vi "PhotonVision_PoseEstData_Alternate.vi"() -> ()   [LabVIEW 2019]
uses:
  <vilib>/Rock Robotics/WPI/ThirdParty/PhotonPoseStrategy_ENUM.ctl
  <vilib>/Rock Robotics/WPI/ThirdParty/PhotonVisionLib/TypeDef/PhotonEstimatedRobotPoseType.ctl
  <vilib>/Rock Robotics/WPI/ThirdParty/JAS_Junk/TrajLib/TypeDef/POSE3D.ctl
  <vilib>/Rock Robotics/WPI/ThirdParty/JAS_Junk/TrajLib/TypeDef/TRANSLATION3D.ctl
  <vilib>/Rock Robotics/WPI/ThirdParty/JAS_Junk/TrajLib/TypeDef/ROTATION3D.ctl
  <vilib>/Rock Robotics/WPI/ThirdParty/JAS_Junk/TrajLib/TypeDef/QUATERNION.ctl
  <vilib>/Rock Robotics/WPI/ThirdParty/PhotonVisionLib/TypeDef/PhotonTrackedTargetType.ctl
  <vilib>/Rock Robotics/WPI/ThirdParty/PhotonVisionLib/TypeDef/TargetCornerType.ctl
  <vilib>/Rock Robotics/WPI/ThirdParty/JAS_Junk/TrajLib/TypeDef/TRANSFORM3D.ctl
  <vilib>/Rock Robotics/WPI/ThirdParty/JAS_Junk/TrajLib/Conv_Deg_Radians.vi
  <vilib>/Rock Robotics/WPI/ThirdParty/JAS_Junk/TrajLib/VI/Quaternion_New.vi
  <vilib>/Rock Robotics/WPI/ThirdParty/JAS_Junk/TrajLib/VI/Transform3d_GetTranslation3d.vi
  <vilib>/Rock Robotics/WPI/ThirdParty/JAS_Junk/TrajLib/VI/Transform3d_GetRotation3d.vi
  <vilib>/Rock Robotics/WPI/ThirdParty/JAS_Junk/TrajLib/VI/Rotation3d_Equals.vi
  <vilib>/Rock Robotics/WPI/ThirdParty/JAS_Junk/TrajLib/VI/Translation3d_Equals.vi
  <vilib>/Rock Robotics/WPI/ThirdParty/PhotonVisionLib/SubVI/PhotonPipelineResult_Unpack.vi
  <vilib>/Rock Robotics/WPI/ThirdParty/PhotonVisionLib/SubVI/PhotonPipelineResult_SetTimeStampSecs.vi
  <vilib>/Rock Robotics/WPI/ThirdParty/PhotonVisionLib/SubVI/PhotonPipelineResult_GetLatency_Millis.vi
  <vilib>/Rock Robotics/WPI/ThirdParty/JAS_Junk/TrajLib/Util_GetTime.vi
  <vilib>/Rock Robotics/WPI/ThirdParty/PhotonVisionLib/SubVI/PhotonPipelineResult_GetTimeStampSecs.vi
  <vilib>/Rock Robotics/WPI/ThirdParty/JAS_Junk/TrajLib/VI/AprilTagFieldLayout_New2022.vi
  <vilib>/Rock Robotics/WPI/ThirdParty/JAS_Junk/TrajLib/VI/AprilTagFieldLayout_New2023.vi
  <vilib>/Rock Robotics/WPI/ThirdParty/JAS_Junk/TrajLib/VI/AprilTagFieldLayout_New2024.vi
  <vilib>/Rock Robotics/WPI/ThirdParty/PhotonVisionLib/SubVI/PhotonTargetModel_New_AprilTag16h5.vi
  <vilib>/Rock Robotics/WPI/ThirdParty/PhotonVisionLib/SubVI/PhotonPoseEstimator_Update_All.vi
  <vilib>/Rock Robotics/WPI/ThirdParty/JAS_Junk/TrajLib/VI/Rotation3d_GetQuaterion.vi
  <vilib>/Rock Robotics/WPI/ThirdParty/JAS_Junk/TrajLib/VI/Quaternion_Equals.vi
  <vilib>/Rock Robotics/WPI/ThirdParty/PhotonVisionLib/SubVI/Packet_decode_Flt64.vi
  <vilib>/Rock Robotics/WPI/ThirdParty/PhotonVisionLib/SubVI/Packet_decode_ByteI8.vi
  <vilib>/Rock Robotics/WPI/ThirdParty/PhotonVisionLib/SubVI/PhotonTrackedTarget_Unpack.vi
  <vilib>/Rock Robotics/WPI/ThirdParty/PhotonVisionLib/SubVI/PhotonMultiTargetPNPResult_unpack.vi
  <vilib>/Rock Robotics/WPI/ThirdParty/PhotonVisionLib/SubVI/PhotonPipelineResult_New.vi
  <vilib>/Rock Robotics/WPI/ThirdParty/JAS_Junk/TrajLib/VI/Util_GetTime_U32.vi
  <vilib>/Rock Robotics/WPI/ThirdParty/JAS_Junk/TrajLib/VI/AprilTagFieldLayout_New.vi
  <vilib>/Rock Robotics/WPI/ThirdParty/JAS_Junk/TrajLib/VI/Pose3d_New_Trans3dRot3d.vi
  <vilib>/Rock Robotics/WPI/ThirdParty/JAS_Junk/TrajLib/VI/Rotation3d_Create_Quaternion.vi
  <vilib>/Rock Robotics/WPI/ThirdParty/JAS_Junk/TrajLib/VI/AprilTag_New.vi
  <vilib>/Rock Robotics/WPI/ThirdParty/PhotonVisionLib/SubVI/PhotonTargetModel_New_RectPlanar.vi
  <vilib>/Rock Robotics/WPI/ThirdParty/JAS_Junk/TrajLib/Conv_Inches_Meters.vi
  <vilib>/Rock Robotics/WPI/ThirdParty/PhotonVisionLib/SubVI/PhotonPoseEstimator_SetLastPose.vi
  <vilib>/Rock Robotics/WPI/ThirdParty/PhotonVisionLib/SubVI/PhotonPoseEstimator_GetEmptyPose.vi
  <vilib>/Rock Robotics/WPI/ThirdParty/PhotonVisionLib/SubVI/PhotonPoseEstimator_lowestAmbiguityStrategy.vi
  <vilib>/Rock Robotics/WPI/ThirdParty/PhotonVisionLib/SubVI/PhotonPoseEstimator_closestToCameraHeightStrategy.vi
  <vilib>/Rock Robotics/WPI/ThirdParty/PhotonVisionLib/SubVI/PhotonPoseEstimator_closestToReferencePoseStrategy.vi
  <vilib>/Rock Robotics/WPI/ThirdParty/PhotonVisionLib/SubVI/PhotonPoseEstimator_GetReferencePose.vi
  <vilib>/Rock Robotics/WPI/ThirdParty/PhotonVisionLib/SubVI/PhotonPoseEstimator_averageBestTargetsStrategy.vi
  <vilib>/Rock Robotics/WPI/ThirdParty/PhotonVisionLib/SubVI/PhotonPoseEstimator_multiTagOnCoprocStrategy.vi
  <vilib>/Rock Robotics/WPI/ThirdParty/JAS_Junk/TrajLib/VI/Quaternion_Get_Vect.vi
  <vilib>/Rock Robotics/WPI/ThirdParty/JAS_Junk/TrajLib/VI/Quaternion_Get_W.vi
  <vilib>/Rock Robotics/WPI/ThirdParty/PhotonVisionLib/SubVI/TargetCorner_New.vi
  <vilib>/Rock Robotics/WPI/ThirdParty/PhotonVisionLib/SubVI/Packet_decode_Int32.vi
  <vilib>/Rock Robotics/WPI/ThirdParty/PhotonVisionLib/SubVI/Packet_decode_Transform3d.vi
  <vilib>/Rock Robotics/WPI/ThirdParty/PhotonVisionLib/SubVI/PhotonPNPResult_unpackt.vi
  <vilib>/Rock Robotics/WPI/ThirdParty/PhotonVisionLib/SubVI/PhotonMultiTargetPNPResult_New.vi
  <vilib>/Rock Robotics/WPI/ThirdParty/PhotonVisionLib/SubVI/PhotonMultiTargetPNPResult_MAX_IDS.vi
  <vilib>/Rock Robotics/WPI/ThirdParty/PhotonVisionLib/SubVI/Packet_decode_Int16.vi
  <vilib>/Rock Robotics/WPI/ThirdParty/JAS_Junk/TrajLib/VI/AprilTag_GetAll.vi
  <vilib>/Rock Robotics/WPI/ThirdParty/JAS_Junk/TrajLib/VI/Quaternion_Normalize.vi
  <vilib>/Rock Robotics/WPI/ThirdParty/PhotonVisionLib/SubVI/PhotonTargetModel_New.vi
  <vilib>/Rock Robotics/WPI/ThirdParty/JAS_Junk/TrajLib/VI/Rotation3d_Create_AxisAngle.vi
  <vilib>/Rock Robotics/WPI/ThirdParty/JAS_Junk/TrajLib/VI/Pose3d_New.vi
  <vilib>/Rock Robotics/WPI/ThirdParty/PhotonVisionLib/SubVI/PhotonPipelineResult_HasTargets.vi
  <vilib>/Rock Robotics/WPI/ThirdParty/PhotonVisionLib/SubVI/PhotonPipelineResult_GetTargets.vi
  <vilib>/Rock Robotics/WPI/ThirdParty/PhotonVisionLib/SubVI/PhotonTrackedTarget_GetPoseAmbiguity.vi
  <vilib>/Rock Robotics/WPI/ThirdParty/PhotonVisionLib/SubVI/PhotonTrackedTarget_GetFiducialId.vi
  <vilib>/Rock Robotics/WPI/ThirdParty/PhotonVisionLib/SubVI/PhotonPoseEstimator_GetFieldTags.vi
  <vilib>/Rock Robotics/WPI/ThirdParty/JAS_Junk/TrajLib/VI/AprilTagFieldLayout_GetTagPose.vi
  <vilib>/Rock Robotics/WPI/ThirdParty/JAS_Junk/TrajLib/VI/Pose3d_TransformBy.vi
  <vilib>/Rock Robotics/WPI/ThirdParty/PhotonVisionLib/SubVI/PhotonTrackedTarget_GetBestCameraToTarget.vi
  <vilib>/Rock Robotics/WPI/ThirdParty/JAS_Junk/TrajLib/VI/Transform3d_Inverse.vi
  <vilib>/Rock Robotics/WPI/ThirdParty/PhotonVisionLib/SubVI/PhotonPoseEstimator_GetRobotToCameraTransform.vi
  <vilib>/Rock Robotics/WPI/ThirdParty/PhotonVisionLib/SubVI/PhotonPoseEstimator_GetHighestAmbiguity.vi
  <vilib>/Rock Robotics/WPI/ThirdParty/PhotonVisionLib/SubVI/PhotonEstimatedRobotPose_New.vi
  <vilib>/Rock Robotics/WPI/ThirdParty/PhotonVisionLib/SubVI/PhotonPoseEstimator_closestToCameraHeightStrategy_calc.vi
  <vilib>/Rock Robotics/WPI/ThirdParty/PhotonVisionLib/SubVI/PhotonTrackedTarget_GetAltCameraToTarget.vi
  <vilib>/Rock Robotics/WPI/ThirdParty/PhotonVisionLib/SubVI/PhotonPoseEstimator_closestToReferencePoseStrategy_calc.vi
  <vilib>/Rock Robotics/WPI/ThirdParty/PhotonVisionLib/SubVI/PhotonPoseEstimator_averageBestTargetsStrategy_calc.vi
  <vilib>/Rock Robotics/WPI/ThirdParty/JAS_Junk/TrajLib/VI/Rotation3d_Plus.vi
  <vilib>/Rock Robotics/WPI/ThirdParty/JAS_Junk/TrajLib/VI/Translation3d_Plus.vi
  <vilib>/Rock Robotics/WPI/ThirdParty/JAS_Junk/TrajLib/VI/Translation3d_Times.vi
  <vilib>/Rock Robotics/WPI/ThirdParty/JAS_Junk/TrajLib/VI/Rotation3d_Times.vi
  <vilib>/Rock Robotics/WPI/ThirdParty/JAS_Junk/TrajLib/VI/Rotation3d_Create_Default.vi
  <vilib>/Rock Robotics/WPI/ThirdParty/JAS_Junk/TrajLib/VI/Translation3d_Create_Default.vi
  <vilib>/Rock Robotics/WPI/ThirdParty/JAS_Junk/TrajLib/VI/Pose3d_New_Default.vi
  <vilib>/Rock Robotics/WPI/ThirdParty/JAS_Junk/TrajLib/VI/Pose3d_Plus.vi
  <vilib>/Rock Robotics/WPI/ThirdParty/JAS_Junk/TrajLib/VI/Pose3d_RelativeTo.vi
  <vilib>/Rock Robotics/WPI/ThirdParty/JAS_Junk/TrajLib/VI/AprilTagFieldLayout_GetOriginPosition.vi
  <vilib>/Rock Robotics/WPI/ThirdParty/PhotonVisionLib/SubVI/PhotonPipelineResult_GetMultiTagResult.vi
  <vilib>/Rock Robotics/WPI/ThirdParty/PhotonVisionLib/SubVI/Packet_decode_Boolean.vi
  <vilib>/Rock Robotics/WPI/ThirdParty/PhotonVisionLib/SubVI/PhotonPNPResult_New_Empty.vi
  <vilib>/Rock Robotics/WPI/ThirdParty/PhotonVisionLib/SubVI/PhotonPNPResult_New.vi
  <vilib>/Rock Robotics/WPI/ThirdParty/JAS_Junk/TrajLib/VI/Quaternion_New_Default.vi
  <vilib>/Rock Robotics/WPI/ThirdParty/JAS_Junk/TrajLib/VI/Vector_Norm.vi
  <vilib>/Rock Robotics/WPI/ThirdParty/JAS_Junk/TrajLib/VecBuilder_ArrayBy1Fill.vi
  <vilib>/Rock Robotics/WPI/ThirdParty/JAS_Junk/TrajLib/VI/Pose3d_getTranslation3d.vi
  <vilib>/Rock Robotics/WPI/ThirdParty/JAS_Junk/TrajLib/VI/Pose3d_getRotation3d.vi
  <vilib>/Rock Robotics/WPI/ThirdParty/JAS_Junk/TrajLib/VI/Translation3d_RotateBy.vi
  <vilib>/Rock Robotics/WPI/ThirdParty/JAS_Junk/TrajLib/VI/Translation3d_ToTranslation2d.vi
  <vilib>/Rock Robotics/WPI/ThirdParty/JAS_Junk/TrajLib/VI/Rotation3d_ToRotation2d.vi
  <vilib>/Rock Robotics/WPI/ThirdParty/JAS_Junk/TrajLib/Transform2d_Create_TransRot.vi
  <vilib>/Rock Robotics/WPI/ThirdParty/JAS_Junk/TrajLib/VI/Rotation3d_UnaryMinus.vi
  <vilib>/Rock Robotics/WPI/ThirdParty/JAS_Junk/TrajLib/VI/Translation3d_UnaryMinus.vi
  <vilib>/Rock Robotics/WPI/ThirdParty/JAS_Junk/TrajLib/VI/Transform3d_GetXYZ.vi
  <vilib>/Rock Robotics/WPI/ThirdParty/JAS_Junk/TrajLib/VI/Pose3d_getXYZ.vi
  <vilib>/Rock Robotics/WPI/ThirdParty/PhotonVisionLib/SubVI/PhotonPoseEstimator_CalcDifference.vi
  <vilib>/Rock Robotics/WPI/ThirdParty/JAS_Junk/TrajLib/VI/Rotation3d_RotateBy.vi
  <vilib>/Rock Robotics/WPI/ThirdParty/JAS_Junk/TrajLib/VI/Translation3d_GetXYZ.vi
  <vilib>/Rock Robotics/WPI/ThirdParty/JAS_Junk/TrajLib/VI/Transform3d_Create_Pose3dPose3d.vi
  <vilib>/Rock Robotics/WPI/ThirdParty/JAS_Junk/TrajLib/MatBuilder_Create.vi
  <vilib>/Rock Robotics/WPI/ThirdParty/JAS_Junk/TrajLib/VI/Quaternion_Times.vi
  <vilib>/Rock Robotics/WPI/ThirdParty/JAS_Junk/TrajLib/VI/Quaternion_Inverse.vi
  <vilib>/Rock Robotics/WPI/ThirdParty/JAS_Junk/TrajLib/VI/Quaternion_Get_All.vi
  <vilib>/Rock Robotics/WPI/ThirdParty/JAS_Junk/TrajLib/Translation2d_Create.vi
  <vilib>/Rock Robotics/WPI/ThirdParty/JAS_Junk/TrajLib/Rotation2d_CreateAngle.vi
  <vilib>/Rock Robotics/WPI/ThirdParty/JAS_Junk/TrajLib/VI/Rotation3d_GetXYZ.vi
  <vilib>/Rock Robotics/WPI/ThirdParty/JAS_Junk/TrajLib/VI/Translation3d_GetDistance.vi
  <vilib>/Rock Robotics/WPI/ThirdParty/JAS_Junk/TrajLib/VI/Translation3d_Minus.vi
  <vilib>/Rock Robotics/WPI/ThirdParty/JAS_Junk/TrajLib/VI/Rotation3d_Minus.vi
  <vilib>/Rock Robotics/Network Tables/NT Write Boolean.vi
  <vilib>/Rock Robotics/Network Tables/NT Read Value.vi
  <vilib>/Rock Robotics/Network Tables/NT Read Raw.vi
  <vilib>/Rock Robotics/SystemInterfaces/Utilities/FPGA_UtilitiesRead LocalTime.vi
  <vilib>/Rock Robotics/WPI/ThirdParty/JAS_Junk/TrajLib/VI/Util_GetTime_U64.vi
  <vilib>/Rock Robotics/WPI/ThirdParty/PhotonVisionLib/PhotonVisionLib.lvlib
  <vilib>/Rock Robotics/WPI/ThirdParty/JAS_Junk/TrajLib/Trajectory_Library.lvlib
panel:
  out "Pos Found 3":bool
  out "Robot Position 3":T1={"EstimatedPose"={"Translation3d"={"X"=0.0, "Y"=0.0, "Z"=0.0}, "Rotation3d"={"Q_quaternion"={"R"=1.0, "V"=[0.0, 0.0, 0.0]}}}, "TimeStamp_Seconds"=0.0, "targetsUsed"=[], "Strategy"=enum."LOWEST_AMBIGUITY"} {"targetsUsed"."AltCameraToTarget"."TRANSLATION3D"."Z" format="%14.3f"; "targetsUsed"."AltCameraToTarget"."TRANSLATION3D"."Y" format="%14.3f"; "targetsUsed"."AltCameraToTarget"."TRANSLATION3D"."X" format="%14.3f"; "targetsUsed"."BestCameraToTarget"."TRANSLATION3D"."Z" format="%14.3f"; "targetsUsed"."BestCameraToTarget"."TRANSLATION3D"."Y" format="%14.3f"; "targetsUsed"."BestCameraToTarget"."TRANSLATION3D"."X" format="%14.3f"; "EstimatedPose"."Translation3d"."Z" format="%14.3f"; "EstimatedPose"."Translation3d"."Y" format="%14.3f"; "EstimatedPose"."Translation3d"."X" format="%14.3f"}
  out "Pos Found 2":bool
  out "Robot Position 2":T1={"EstimatedPose"={"Translation3d"={"X"=0.0, "Y"=0.0, "Z"=0.0}, "Rotation3d"={"Q_quaternion"={"R"=1.0, "V"=[0.0, 0.0, 0.0]}}}, "TimeStamp_Seconds"=0.0, "targetsUsed"=[], "Strategy"=enum."LOWEST_AMBIGUITY"} {"targetsUsed"."AltCameraToTarget"."TRANSLATION3D"."Z" format="%14.3f"; "targetsUsed"."AltCameraToTarget"."TRANSLATION3D"."Y" format="%14.3f"; "targetsUsed"."AltCameraToTarget"."TRANSLATION3D"."X" format="%14.3f"; "targetsUsed"."BestCameraToTarget"."TRANSLATION3D"."Z" format="%14.3f"; "targetsUsed"."BestCameraToTarget"."TRANSLATION3D"."Y" format="%14.3f"; "targetsUsed"."BestCameraToTarget"."TRANSLATION3D"."X" format="%14.3f"; "EstimatedPose"."Translation3d"."Z" format="%14.3f"; "EstimatedPose"."Translation3d"."Y" format="%14.3f"; "EstimatedPose"."Translation3d"."X" format="%14.3f"}
  in  "Strategy 3":T9=enum."AVERAGE_BEST_TARGETS"
  in  "Strategy 2":T9
  out "Pipeline HasTargets":bool
  in  "Yaw  Degrees":dbl format="%#_13g"
  in  "Pitch  Degrees":dbl format="%#_13g"
  in  "Roll  Degrees":dbl format="%#_13g"
  in  "Z Meters":dbl=0.8 format="%#_13g"
  in  "Y Meters":dbl format="%#_13g"
  in  "X Meters":dbl format="%#_13g"
  in  "Highest\nAllowed \nAmbiguity":dbl=10.0
  out "New Data":bool
  out "Pos Found 1":bool
  out "Robot Position 1":T1={"EstimatedPose"={"Translation3d"={"X"=0.0, "Y"=0.0, "Z"=0.0}, "Rotation3d"={"Q_quaternion"={"R"=1.0, "V"=[0.0, 0.0, 0.0]}}}, "TimeStamp_Seconds"=0.0, "targetsUsed"=[], "Strategy"=enum."LOWEST_AMBIGUITY"} {"targetsUsed"."AltCameraToTarget"."TRANSLATION3D"."Z" format="%14.3f"; "targetsUsed"."AltCameraToTarget"."TRANSLATION3D"."Y" format="%14.3f"; "targetsUsed"."AltCameraToTarget"."TRANSLATION3D"."X" format="%14.3f"; "targetsUsed"."BestCameraToTarget"."TRANSLATION3D"."Z" format="%14.3f"; "targetsUsed"."BestCameraToTarget"."TRANSLATION3D"."Y" format="%14.3f"; "targetsUsed"."BestCameraToTarget"."TRANSLATION3D"."X" format="%14.3f"; "EstimatedPose"."Translation3d"."Z" format="%14.3f"; "EstimatedPose"."Translation3d"."Y" format="%14.3f"; "EstimatedPose"."Translation3d"."X" format="%14.3f"}
  in  "AprilTagField":enum16{"2022 Rapid React", "2023 Charged Up"}(ring)=enum."2023 Charged Up"
  in  "Strategy 1":T9=enum."CLOSEST_TO_LAST_POSE"
  out "IsConnected":bool
  in  "CameraName":string="Microsoft LifeCam HD-3000"
  out "Loop Count":i32
  # "Camera Position On Robot"
  # "Suggest never selecting the \"CLOSEST_TO_LAST_POSE\"\nfor Strategy 2 or Strategy 3.  Only Strategy 1 data is fed\nback from the previous execution cycle.  In other words\nthe Last Pose is never saved for Strategy or Strategy 3."
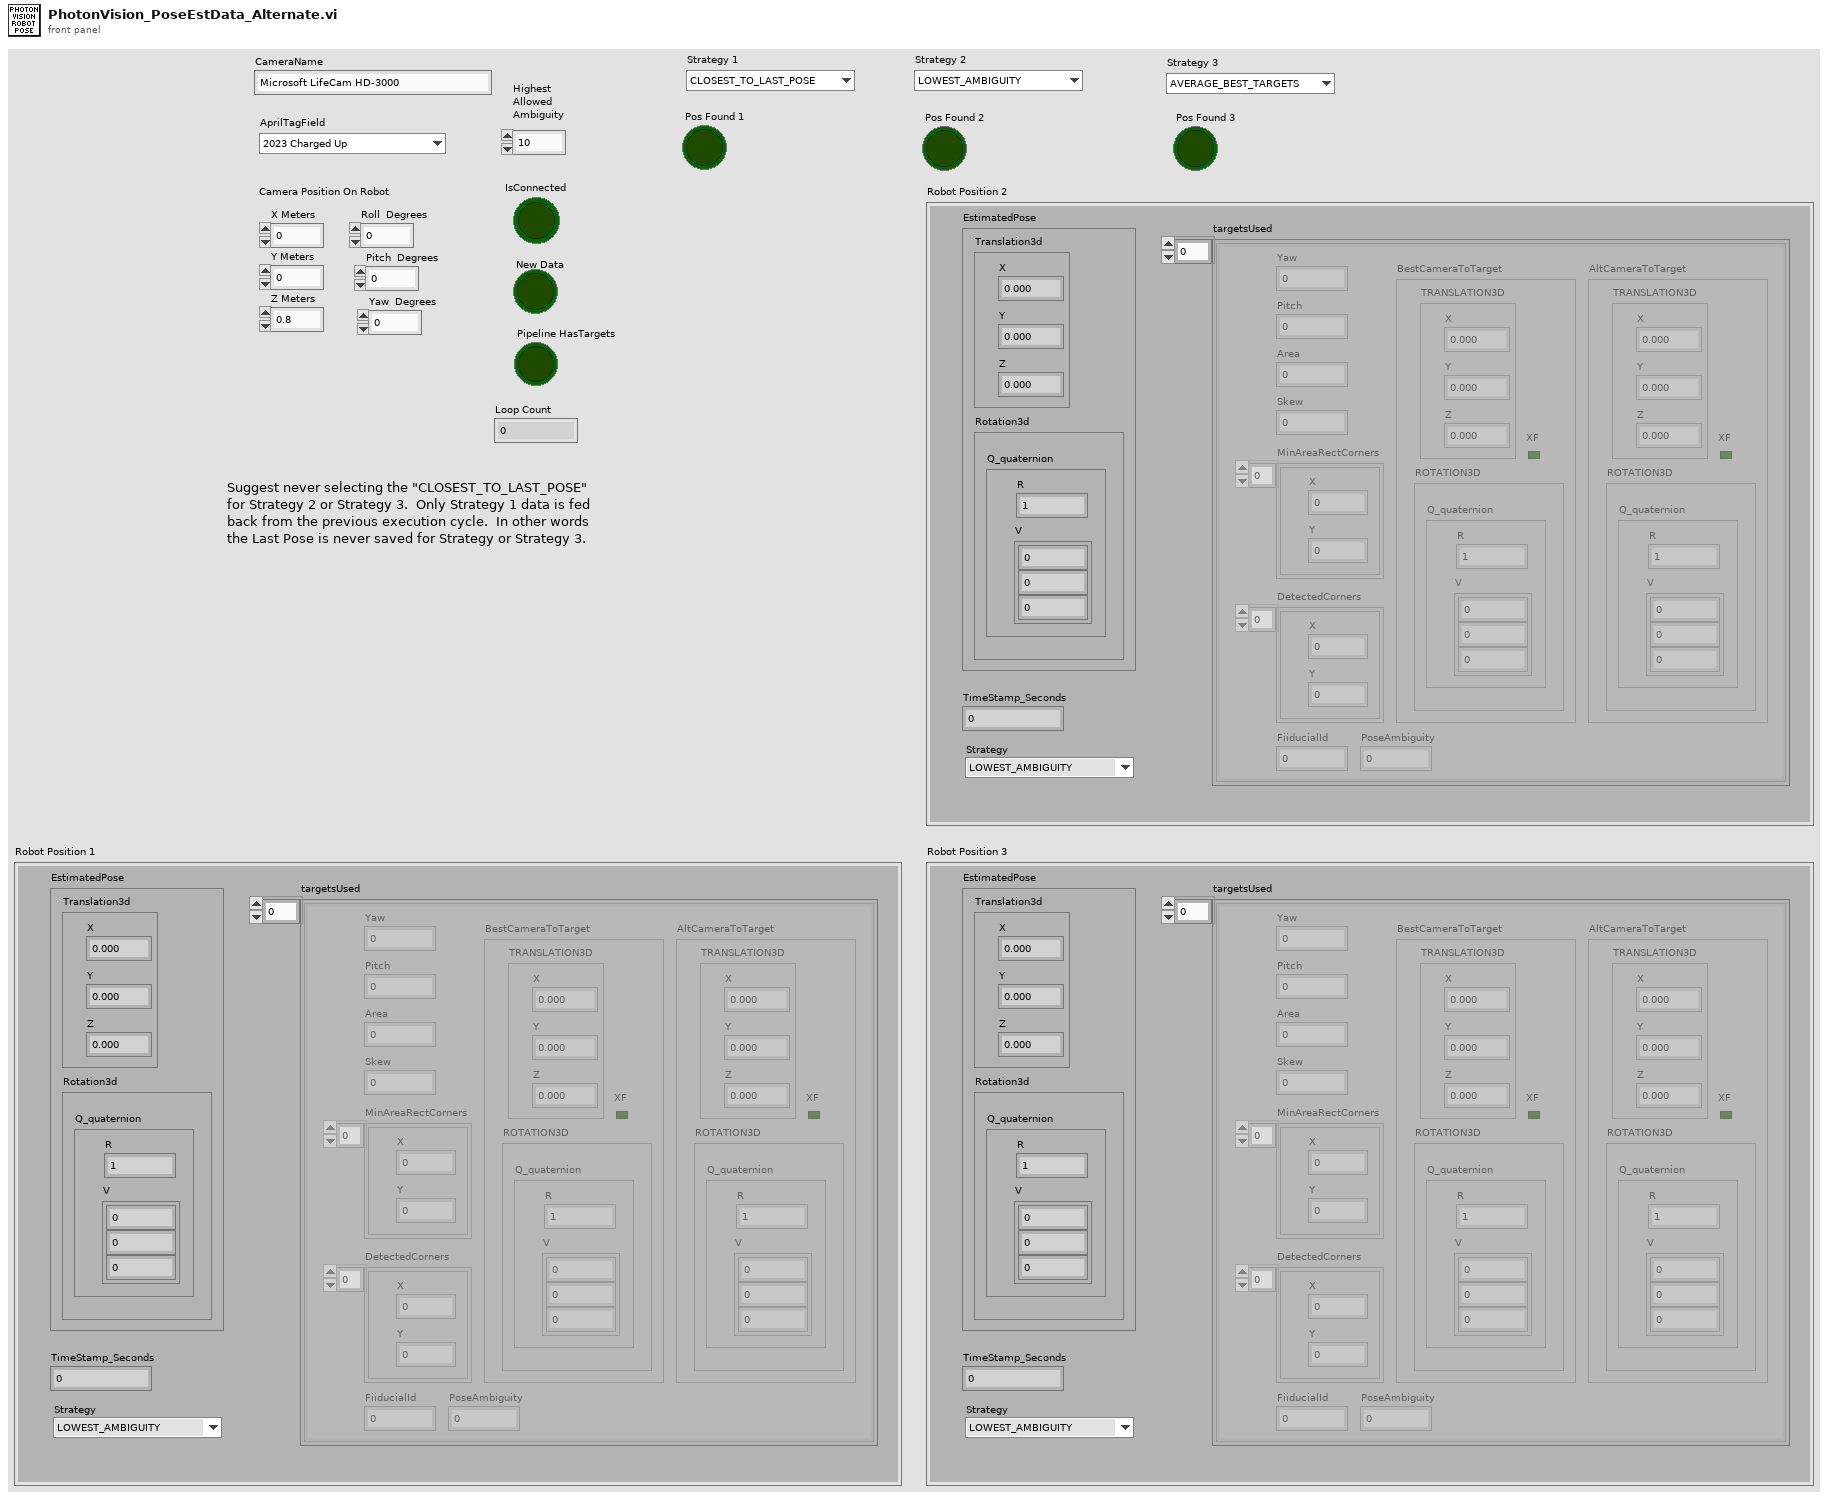
[diagram p1: front panel]
types:
  T1 = typedef "PhotonVisionLib.lvlib/PhotonEstimatedRobotPoseType.ctl" = cluster{"EstimatedPose":T2, "TimeStamp_Seconds":dbl, "targetsUsed":T6[], "Strategy":T9}
  T2 = typedef "Trajectory_Library.lvlib/POSE3D.ctl" = cluster{"Translation3d":T3, "Rotation3d":T4}
  T3 = typedef "Trajectory_Library.lvlib/TRANSLATION3D.ctl" = cluster{"X":dbl, "Y":dbl, "Z":dbl}
  T4 = typedef "Trajectory_Library.lvlib/ROTATION3D.ctl" = cluster{"Q_quaternion":T5}
  T5 = typedef "Trajectory_Library.lvlib/QUATERNION.ctl" = cluster{"R":dbl, "V":dbl[]}
  T6 = typedef "PhotonVisionLib.lvlib/PhotonTrackedTargetType.ctl" = cluster{"Yaw":dbl, "Pitch":dbl, "Area":dbl, "Skew":dbl, "MinAreaRectCorners":T7[], "BestCameraToTarget":T8, "FiiducialId":i32, "AltCameraToTarget":T8, "PoseAmbiguity":dbl, "DetectedCorners":T7[]}
  T7 = typedef "PhotonVisionLib.lvlib/TargetCornerType.ctl" = cluster{"X":dbl, "Y":dbl}
  T8 = typedef "Trajectory_Library.lvlib/TRANSFORM3D.ctl" = cluster{"TRANSLATION3D":T3, "ROTATION3D":T4, "XF":bool}
  T9 = typedef "PhotonVisionLib.lvlib/PhotonPoseStrategy_ENUM.ctl" = enum16{"LOWEST_AMBIGUITY", "CLOSEST_TO_CAMERA_HEIGHT", "CLOSEST_TO_REFERENCE_POSE", "CLOSEST_TO_LAST_POSE", "AVERAGE_BEST_TARGETS", "MULTI_TAG_PNP_ON_COPROCESSOR", "MULTI_TAG_PNP_ON_RIO"}
  T10 = typedef "Trajectory_Library.lvlib/AprilTagFieldLayout.ctl" = cluster{"AprilTagMap":map{i32, T11}, "FieldLength":dbl, "FieldWidth":dbl, "OriginPosition ":T12, "OriginPose3d":T2}
  T11 = typedef "Trajectory_Library.lvlib/AprilTag.ctl" = cluster{"ID":i32, "POSE3D":T2}
  T12 = typedef "Trajectory_Library.lvlib/AprilTagFieldLayoutOrignPosition_ENUM.ctl" = enum16{"kBlueAllianceWallRightSide,", "kRedAllianceWallRightSide,"}
  T13 = typedef "PhotonVisionLib.lvlib/PhotonPoseEstimatorType.ctl" = cluster{"LastPose":T2, "ReferencePose":T2, "FieldTags":T10, "PrimaryStratety":T9, "Camera":string, "RobotToCamera":T8, "ReportedErrors":dbl[], "HighestAmbiguity":dbl, "MultiTagFallbackStrategy":T9, "PoseCacheTimeoutSec":dbl, "PhotonTargetModel":T14, "BaseNTName":string}
  T14 = typedef "PhotonVisionLib.lvlib/PhotonTargetModel.ctl" = cluster{"Vertices":T3[], "IsPlaner":bool, "IsSpherical":bool}
  T15 = typedef "PhotonVisionLib.lvlib/PhotonPipelineResultType.ctl" = cluster{"TargetCount":i32, "Latency_MilliSec":dbl, "Targets":T6[], "TimeStampSec":dbl, "PhotonMultiTargetPNPResult":T16}
  T16 = typedef "PhotonVisionLib.lvlib/PhotonMultiTargetPNPResultType.ctl" = cluster{"PhotonPNPResult":T17, "FiducialIDsUsed":i16[]}
  T17 = typedef "PhotonVisionLib.lvlib/PhotonPNPResultType.ctl" = cluster{"IsPresent":bool, "bestReprojErr":dbl, "altReprojErr":dbl, "ambiguity":dbl, "Best":T8, "Alt":T8}
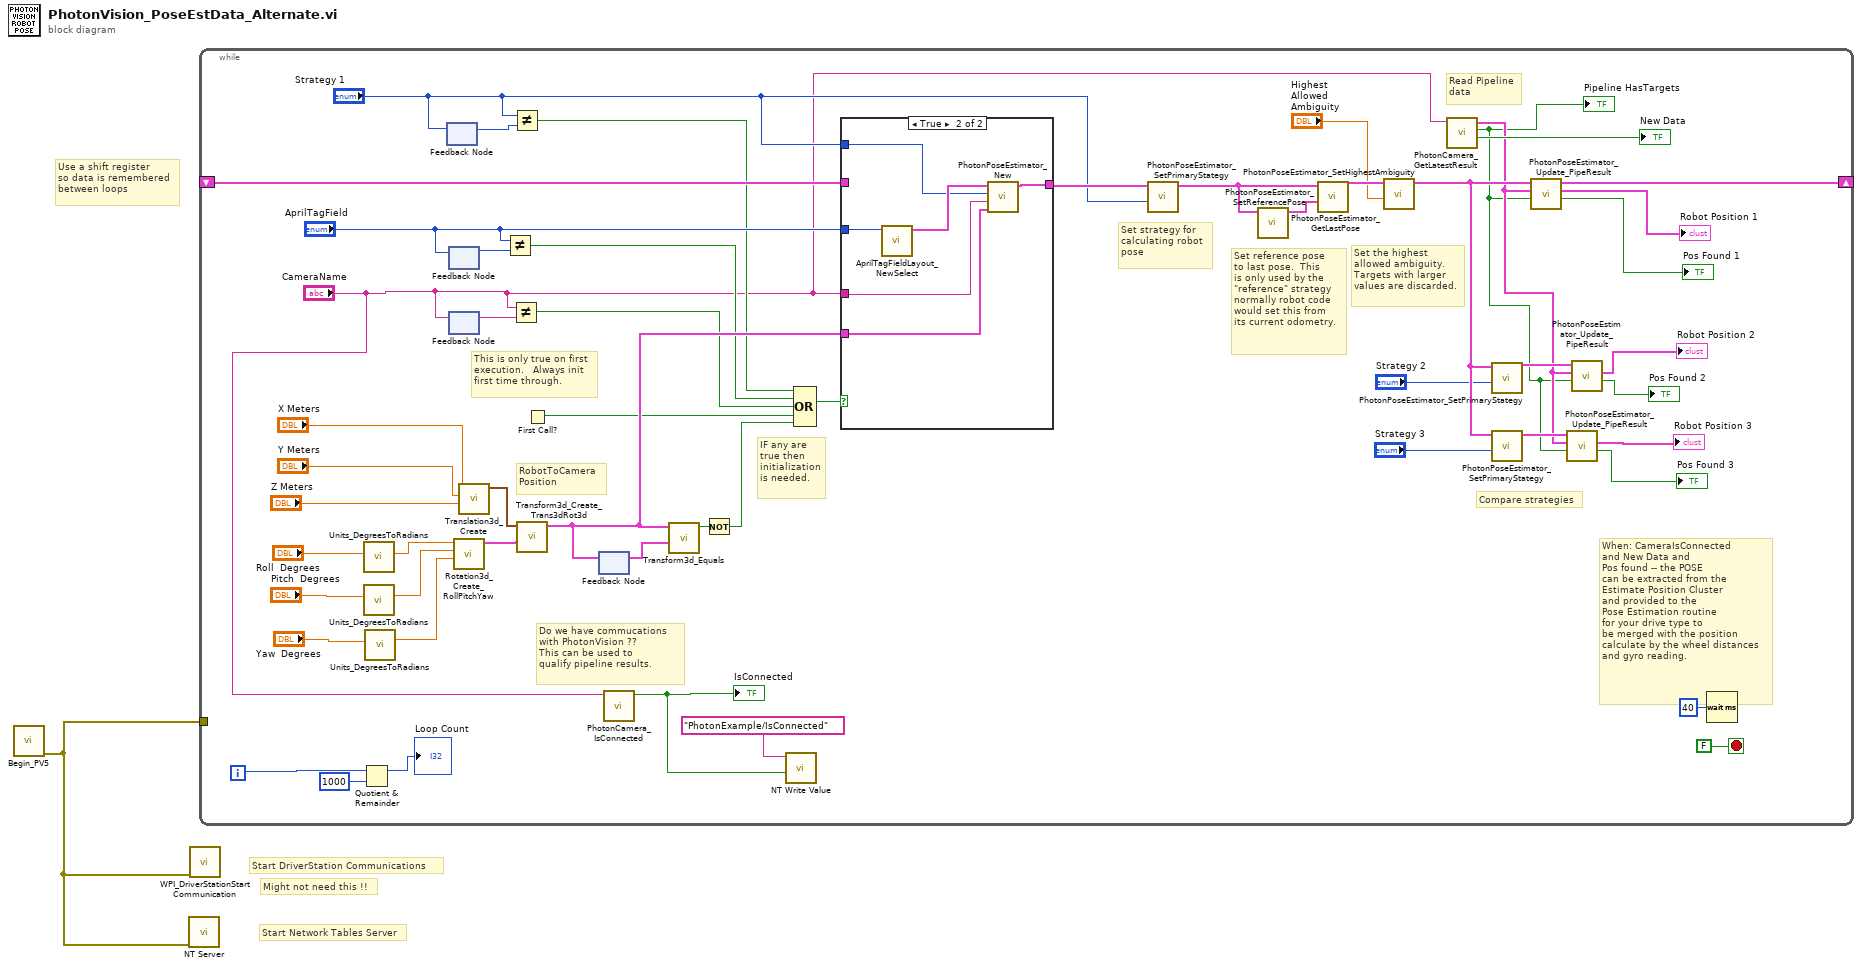
[diagram p0: block diagram]
diagram:
  # "Use a shift register\nso data is remembered\nbetween loops"
  # "Might not need this !!"
  # "Start Network Tables Server"
  # "Start DriverStation Communications"
  n1 = call "Begin_PV5.vi"() -> ("error out"=w1:errorcluster)  [unwired: 11 in]
  n2 = call <vilib>:"NT Server.vi"("error in (no error)"=w1) -> ()  [unwired: 11 in]
  n3 = call <vilib>:"WPI_DriverStationStart Communication.vi"("error in (no error)"=w1) -> ()  [unwired: 11 in]
  n4 = while {
    tunnel: w1 -> [_]
    shift-right: [w16] -> _
    shift-left: _ -> [w47]
    i -> [w53]
    stop <- FALSE stop-if-true
    # "When: CameraIsConnected\nand New Data and\nPos found -- the POSE\ncan be extracted from the\nEstimate Position Cluster\nand provided to the \nPose Estimation routine\nfor your drive type to\nbe merged with the position\ncalculate by the wheel distances\nand gyro reading."
    # "Compare strategies"
    # "Read Pipeline\ndata"
    # "IF any are\ntrue then\ninitialization\nis needed."
    # "This is only true on first\nexecution.   Always init\nfirst time through."
    # "Set the highest\nallowed ambiguity.\nTargets with larger\nvalues are discarded."
    # "Set reference pose\nto last pose.  This\nis only used by the\n\"reference\" strategy\nnormally robot code\nwould set this from\nits current odometry."
    # "Set strategy for\ncalculating robot\npose"
    # "RobotToCamera\nPosition"
    # "Do we have commucations\nwith PhotonVision ??\nThis can be used to\nqualify pipeline results."
    n5 = Quotient & Remainder(x=w53, y=1000) -> (x-y*floor(x/y)=→"Loop Count":i32)  [unwired: 1 out]
    n6 = call <vilib>:"Units_DegreesToRadians.vi"("Degrees"="Roll  Degrees") -> ("Radians"=w44:dbl)  [unwired: 10 in]
    n7 = call <vilib>:"Units_DegreesToRadians.vi"("Degrees"="Pitch  Degrees") -> ("Radians"=w43:dbl)  [unwired: 10 in]
    n8 = call <vilib>:"Units_DegreesToRadians.vi"("Degrees"="Yaw  Degrees") -> ("Radians"=w42:dbl)  [unwired: 10 in]
    n9 = feedback-in #1("Strategy 1") -> ()
    n10 = feedback #1() -> (w30:T9)  [unwired: 1 in]
    n11 = feedback #2() -> (w28:enum16{"2022 Rapid React", "2023 Charged Up"})  [unwired: 1 in]
    n12 = feedback-in #2("AprilTagField") -> ()
    n13 = feedback #3() -> (w27:string)  [unwired: 1 in]
    n14 = feedback-in #3("CameraName") -> ()
    n15 = call <vilib>:"Rotation3d_Create_RollPitchYaw.vi"("Yaw"=w42, "Pitch"=w43, "Roll"=w44) -> ("Rotation3d"=w45:T4)  [unwired: 8 in]
    n16 = call <vilib>:"Translation3d_Create.vi"("Z"="Z Meters", "Y"="Y Meters", "X"="X Meters") -> ("TRANSLATION3D"=w46:T3)  [unwired: 8 in]
    n17 = Not Equal?(x="AprilTagField", y=w28) -> (x != y?=w21:bool)
    n18 = Not Equal?(x="CameraName", y=w27) -> (x != y?=w20:bool)
    n19 = Not Equal?(x="Strategy 1", y=w30) -> (x != y?=w22:bool)
    n20 = call <vilib>:"Transform3d_Create_Trans3dRot3d.vi"("Rotation3d"=w45, "Translation3d"=w46) -> ("Transform3d"=w25:T8)  [unwired: 9 in]
    n21 = First Call?() -> (First Call?: T/F=w19:bool)
    n22 = feedback #4() -> (w24:T8)  [unwired: 1 in]
    n23 = feedback-in #4(w25) -> ()
    n24 = call <vilib>:"PhotonCamera_IsConnected.vi"("CameraName"="CameraName") -> ("IsConnected"=w49:bool)  [unwired: 9 in, 1 out]
    "IsConnected" <- w49
    n25 = call <vilib>:"Transform3d_Equals.vi"("otherTransform3d"=w24, "inTransform3d"=w25) -> ("Equals"=w23:bool)  [unwired: 9 in]
    n26 = Not(x=w23) -> (.not. x?=w18:bool)
    n27 = call-poly <vilib>:"NT Write Value.vi"("Boolean"=w49, "Name"="PhotonExample/IsConnected") -> ()  [unwired: 9 in, 1 out]
    n28 = Compound Arithmetic op=OR(w22, w21, w20, w19, w18) -> (w26:bool)
    n29 = case shown="True" w26 {
      tunnel: [w56 w62] -> w48
      tunnel: "AprilTagField" -> [_ w61]
      tunnel: "CameraName" -> [_ w59]
      tunnel: w47 -> [w56 _]
      tunnel: "Strategy 1" -> [_ w58]
      tunnel: w25 -> [_ w57]
      frame False {
      }
      frame True {
        n30 = call <vilib>:"AprilTagFieldLayout_NewSelect.vi"("AprilTagField"=w61) -> ("AprilTagFieldLayout"=w60:T10)  [unwired: 10 in]
        n31 = call <vilib>:"PhotonPoseEstimator_New.vi"("RobotToCamera"=w57, "Camera"=w59, "Strategy"=w58, "AprilTagFieldLayout"=w60) -> ("PhotonPoseEstimator"=w62:T13)  [unwired: 7 in]
      }
    }
    n32 = call <vilib>:"PhotonPoseEstimator_SetPrimaryStategy.vi"("PrimaryStrategy"="Strategy 1", "PhotonPoseEstimator"=w48) -> ("out PhotonPoseEstimator"=w34:T13)  [unwired: 9 in]
    n33 = call <vilib>:"PhotonPoseEstimator_GetLastPose.vi"("PhotonPoseEstimator"=w34) -> ("LastPose"=w35:T2)  [unwired: 10 in]
    n34 = call <vilib>:"PhotonPoseEstimator_SetReferencePose.vi"("ReferencePose"=w35, "PhotonPoseEstimator"=w34) -> ("out PhotonPoseEstimator"=w33:T13)  [unwired: 9 in]
    n35 = call <vilib>:"PhotonPoseEstimator_SetHighestAmbiguity.vi"("HighestAmbiguity"="Highest\nAllowed \nAmbiguity", "PhotonPoseEstimator"=w33) -> ("out PhotonPoseEstimator"=w14:T13)  [unwired: 9 in]
    n36 = call <vilib>:"PhotonCamera_GetLatestResult.vi"("CameraName"="CameraName") -> ("New Data"=→"New Data":bool, "HasTargets"=w6:bool, "PipelineResult"=w7:T15)  [unwired: 7 in, 1 out]
    "Pipeline HasTargets" <- w6
    n37 = call <vilib>:"PhotonPoseEstimator_SetPrimaryStategy.vi"("PrimaryStrategy"="Strategy 2", "PhotonPoseEstimator"=w14) -> ("out PhotonPoseEstimator"=w9:T13)  [unwired: 9 in]
    n38 = call <vilib>:"PhotonPoseEstimator_SetPrimaryStategy.vi"("PrimaryStrategy"="Strategy 3", "PhotonPoseEstimator"=w14) -> ("out PhotonPoseEstimator"=w8:T13)  [unwired: 9 in]
    n39 = call <vilib>:"PhotonPoseEstimator_Update_PipeResult.vi"("Has Results"=w6, "PipelineResult"=w7, "PhotonPoseEstimator"=w14) -> ("Pos Found"=→"Pos Found 1":bool, "PhotonEstimatedRobotPose"=→"Robot Position 1":T1, "out PhotonPoseEstimator"=w16:T13)  [unwired: 6 in]
    n40 = call <vilib>:"PhotonPoseEstimator_Update_PipeResult.vi"("Has Results"=w6, "PipelineResult"=w7, "PhotonPoseEstimator"=w8) -> ("Pos Found"=→"Pos Found 3":bool, "PhotonEstimatedRobotPose"=→"Robot Position 3":T1)  [unwired: 6 in, 1 out]
    n41 = call <vilib>:"PhotonPoseEstimator_Update_PipeResult.vi"("Has Results"=w6, "PipelineResult"=w7, "PhotonPoseEstimator"=w9) -> ("Pos Found"=→"Pos Found 2":bool, "PhotonEstimatedRobotPose"=→"Robot Position 2":T1)  [unwired: 6 in, 1 out]
    n42 = Wait (ms)(milliseconds to wait=u32 40) -> ()  [unwired: 1 out]
  }
